vi "Shooter logic.vi"(0 "Low Pressure?":bool, 1 "Fire Main":bool, 2 "Fire 3":bool, 3 "Fire 2":bool, 5 "Grabber Button":bool, 6 "Time Between Open and Shoot":u32=250, 7 "Arms Up button":bool, 8 "Release to Retract":u32=750, 9 "Arms Down Button":bool, 10 "Arms up and down":dbl) -> ()   [LabVIEW 2013]
uses:
  <vilib>/Rock Robotics/WPI/Solenoid/WPI_SolenoidValue.ctl
  <vilib>/Rock Robotics/WPI/Solenoid/WPI_SolenoidSetEnum.vi
  Robot Global Data.vi
panel:
  in  "Bottom Limit":dbl
  in  "Top Limit":dbl
  in  "Potientiometer?":bool
  out "Voltage":dbl
  in  "Arm State":enum16{"Close Arms", "Open Arms"}(ring)
  in  "Launcher State":T1(ring)=enum."Retract"
  out "Tick":u32
  out "Retract Position":T2
  out "Shooter Position":T2
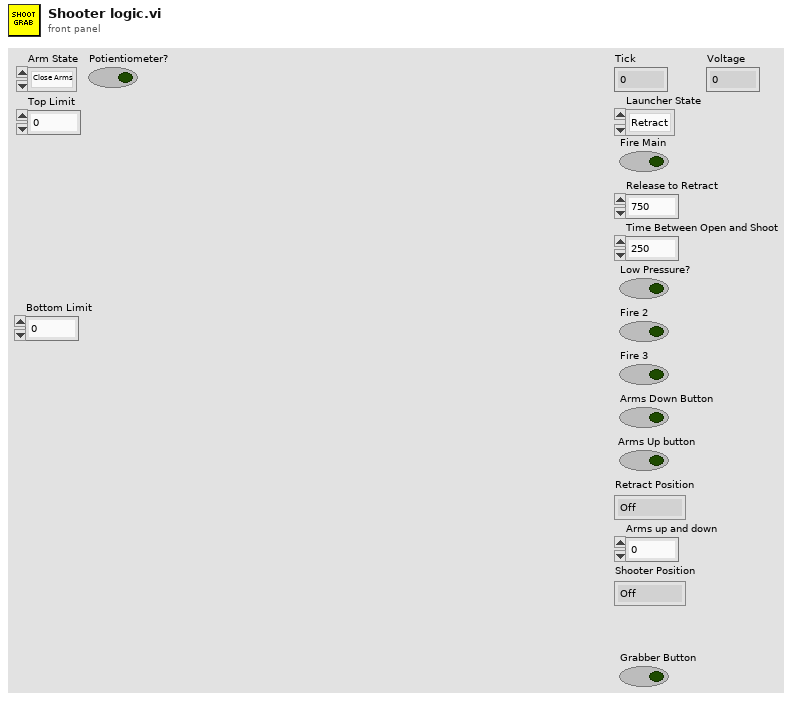
[diagram p1: front panel]
types:
  T1 = enum16{"Open Arms", "Arms Open", "Shoot", "Out", "Retract"}
  T2 = typedef "WPI_SolenoidValue.ctl" = enum16{"Off", "On", "Forward", "Reverse"}
  T3 = typedef "WPI_DigitalInputDevRef.ctl" = cluster{"DevStatus":errorcluster, "DIO Channel":T4, "Digital Module":T5}
  T4 = typedef "FPGA_DIOChannel.ctl" = enum8{"DIO 1", "DIO 2", "DIO 3", "DIO 4", "DIO 5", "DIO 6", "DIO 7", "DIO 8", "DIO 9", "DIO 10", "DIO 11", "DIO 12", "DIO 13", "DIO 14", "Invalid"}
  T5 = typedef "FPGA_TypedefDigitalModule.ctl" = enum16{"Digital Module 1", "Digital Module 2"}
  T6 = typedef "WPI_SolenoidDevRef.ctl" = cluster{"DevStatus":errorcluster, "Solenoid Module":T7, "Forward Solenoid Channel":T8, "Reverse Solenoid Channel":T8}
  T7 = typedef "FPGA_TypedefSolenoidModule.ctl" = enum16{"Solenoid Module 1", "Solenoid Module 2"}
  T8 = typedef "WPI_SolenoidChannel.ctl" = enum8{"Solenoid 1", "Solenoid 2", "Solenoid 3", "Solenoid 4", "Solenoid 5", "Solenoid 6", "Solenoid 7", "Solenoid 8", "Invalid"}
  T9 = typedef "WPI_AnalogChannelDevRef.ctl" = cluster{"DevStatus":errorcluster, "Analog Module":T10, "Analog Channel":T11}
  T10 = typedef "FPGA_TypedefAnalogModule.ctl" = enum16{"Analog Module 1", "Analog Module 2"}
  T11 = typedef "FPGA_AIChannel.ctl" = enum8{"AI 1", "AI 2", "AI 3", "AI 4", "AI 5", "AI 6", "AI 7", "AI 8", "Invalid"}
  T12 = typedef "WPI_MotorControlDeviceRef.ctl" = cluster{"DeviceStatus":errorcluster, "Type":enum16{"PWM", "CAN"}, "PWM":cluster{"Digital Module":T5, "PWM Channel":T13, "DeadBand":T14}, "CAN":cluster{"Device Number":u8, "Control Mode":T15, "Semaphore":T16, "Max Vout":dbl}, "Invert":bool, "TransformRef":T17, "InvTransformRef":T17}
  T13 = typedef "FPGA_DIOPWMChannel.ctl" = enum8{"PWM 1", "PWM 2", "PWM 3", "PWM 4", "PWM 5", "PWM 6", "PWM 7", "PWM 8", "PWM 9", "PWM 10", "Invalid"}
  T14 = typedef "WPI_PWMDeadband.ctl" = cluster{"Name":string, "maxPositivePwm":i32, "minPositivePwm":i32, "centerPwm":i32, "maxNegativePwm":i32, "minNegativePwm":i32, "angularRange":u16}
  T15 = typedef "WPI_CANJaguar_ControlMode.ctl" = enum8{"Percent VBus", "Current", "Speed", "Position", "Voltage"}
  T16 = typedef "Semaphore RefNum" = refnum<k1>
  T17 = typedef "WPI_PWMTransform_ConPane.ctl" = refnum<vi>
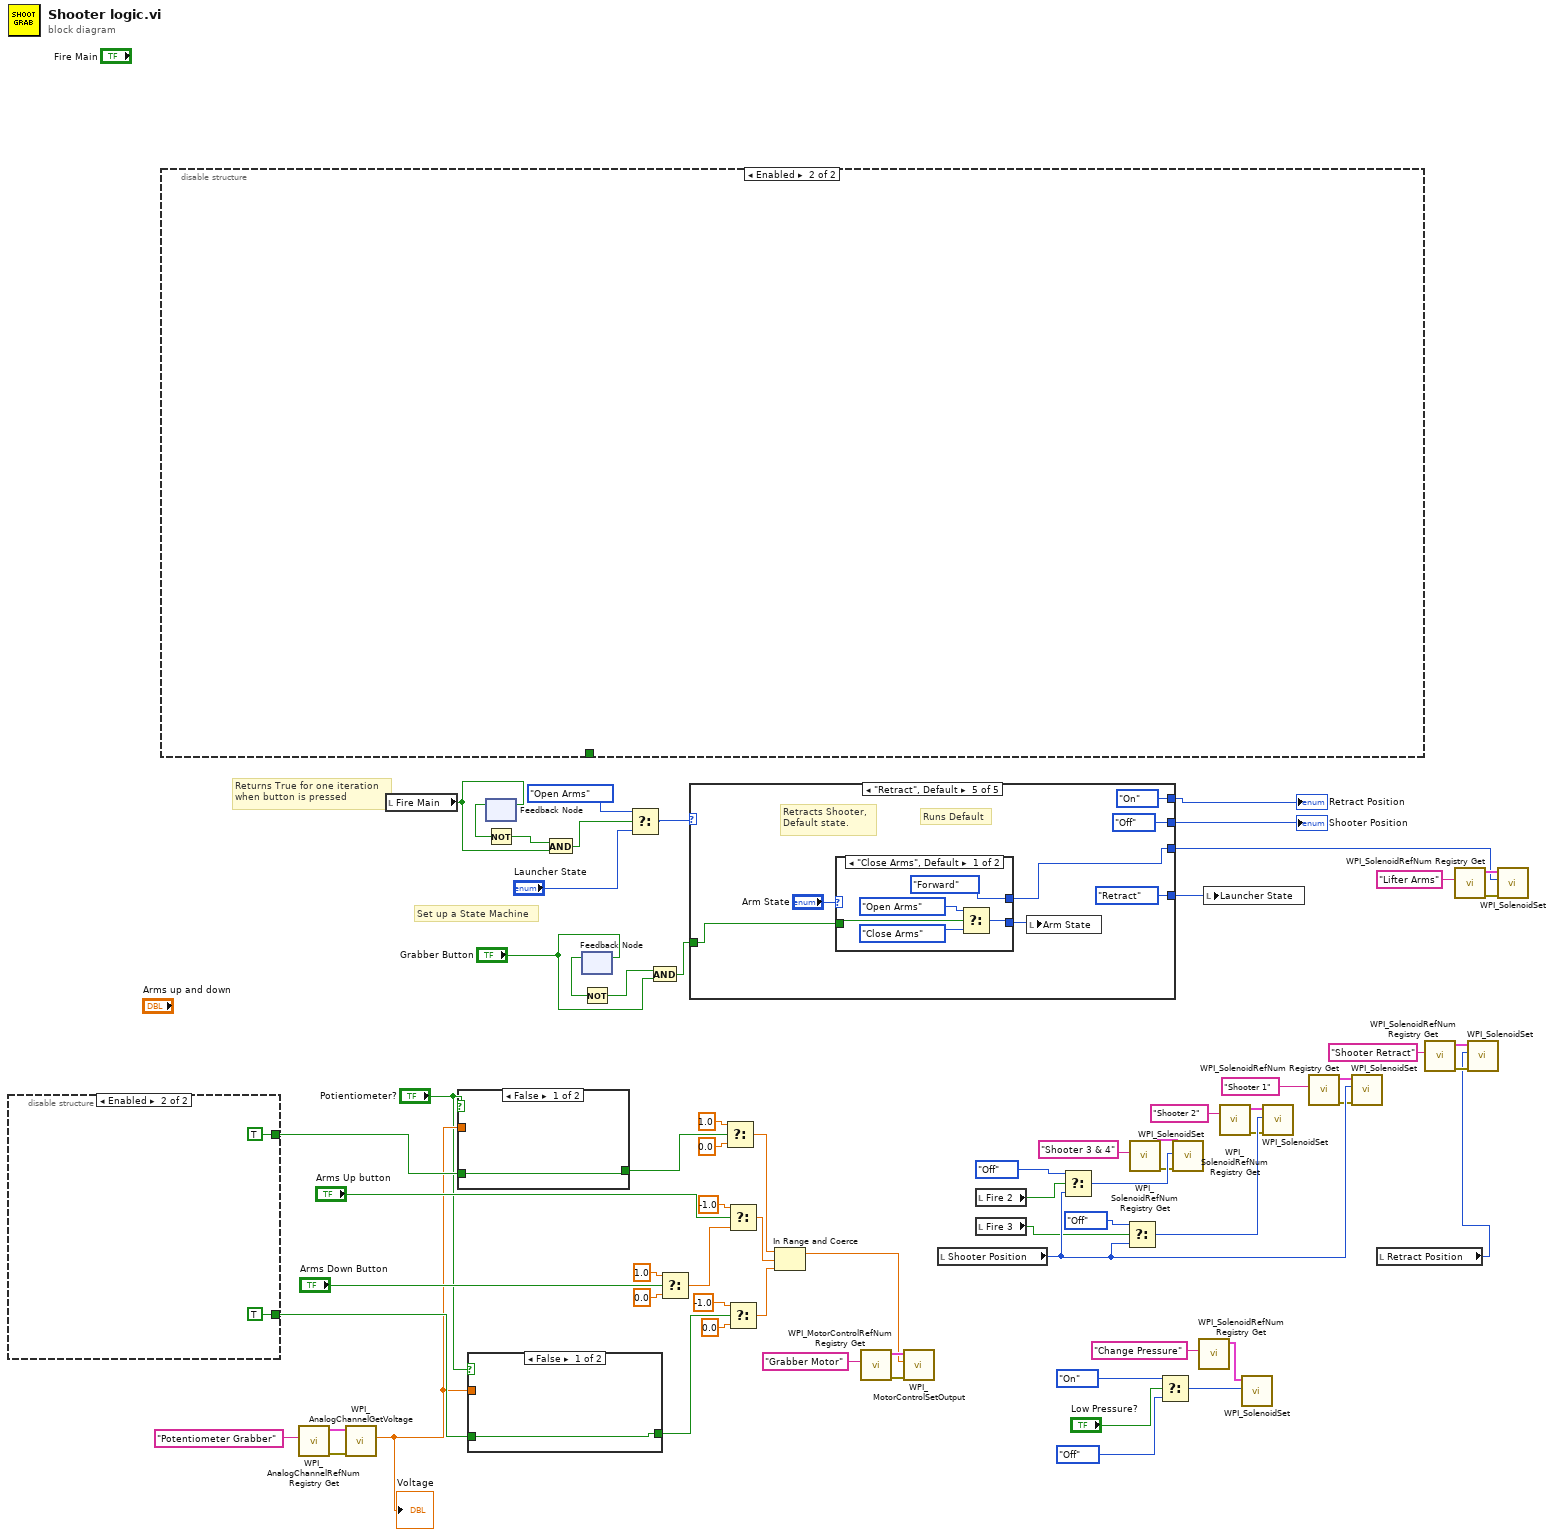
[diagram p0: block diagram]
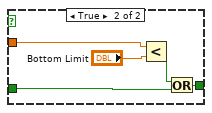
[diagram p2: hidden frame]
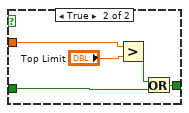
[diagram p3: hidden frame]
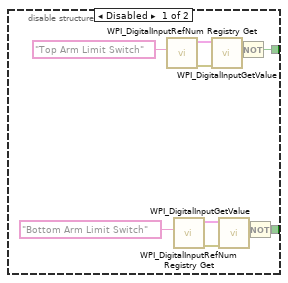
[diagram p4: hidden frame]
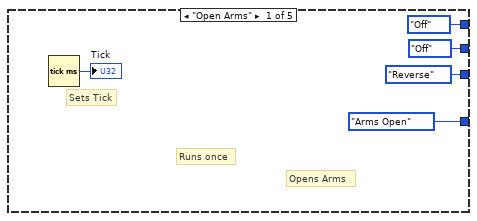
[diagram p5: hidden frame]
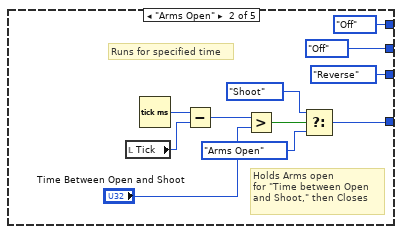
[diagram p6: hidden frame]
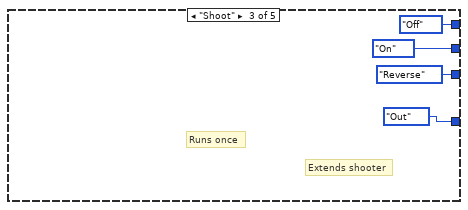
[diagram p7: hidden frame]
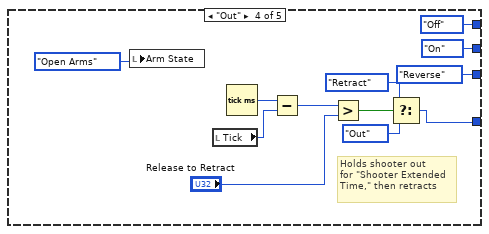
[diagram p8: hidden frame]
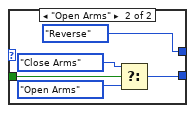
[diagram p9: hidden frame]
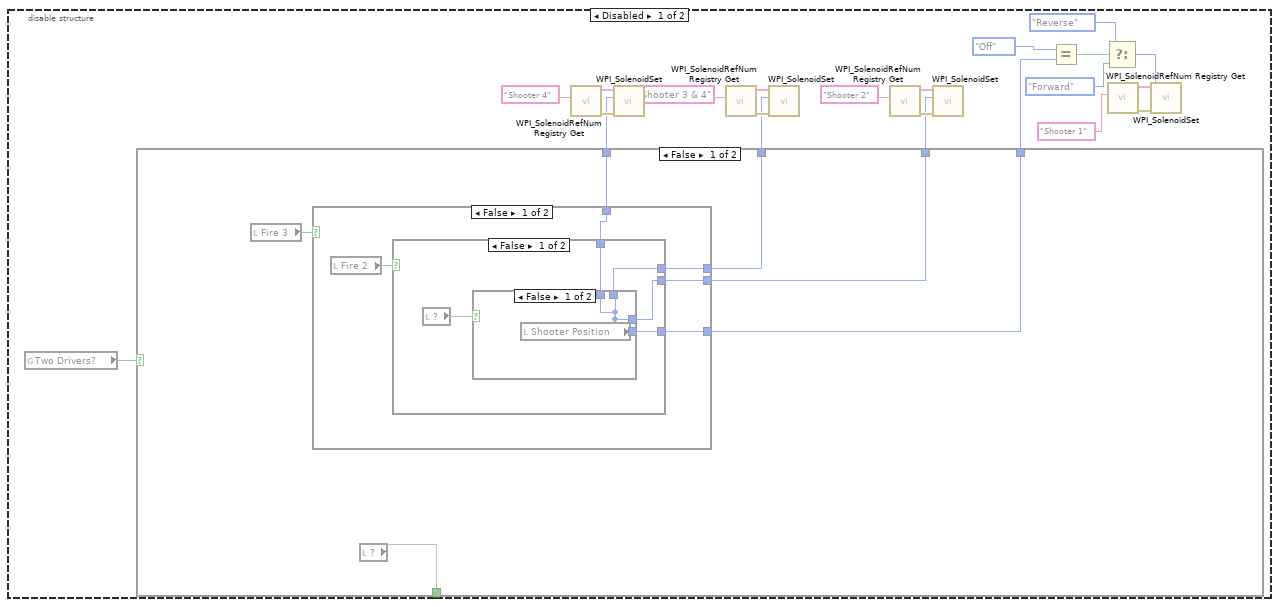
[diagram p10: hidden frame]
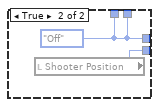
[diagram p11: hidden frame]
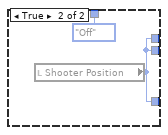
[diagram p12: hidden frame]
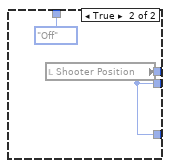
[diagram p13: hidden frame]
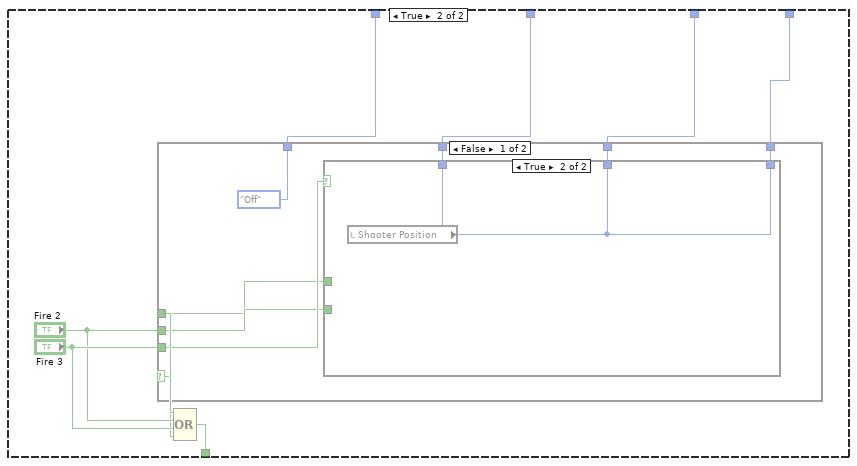
[diagram p14: hidden frame]
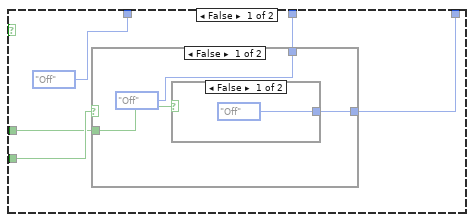
[diagram p15: hidden frame]
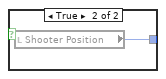
[diagram p16: hidden frame]
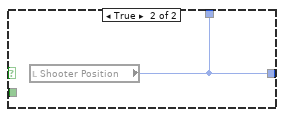
[diagram p17: hidden frame]
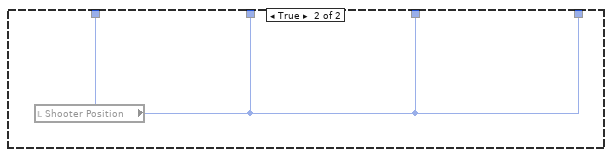
[diagram p18: hidden frame]
diagram:
  # "Set up a State Machine"
  # "Returns True for one iteration\nwhen button is pressed"
  n1 = disable-structure shown="Enabled" {
    disable-tunnel: [w72 TRUE ("Value")] -> w5
    disable-tunnel: [w71 TRUE ("Value")] -> w4
    frame Disabled {
      n2 = call <vilib>:"WPI_DigitalInputRefNum Registry Get.vi"("refnum name"="Top Arm Limit Switch") -> ("error out"=w78:errorcluster, "DigitalInputDevRef"=w79:T3)  [unwired: 9 in]
      n3 = call <vilib>:"WPI_DigitalInputRefNum Registry Get.vi"("refnum name"="Bottom Arm Limit Switch") -> ("error out"=w75:errorcluster, "DigitalInputDevRef"=w76:T3)  [unwired: 9 in]
      n4 = call <vilib>:"WPI_DigitalInputGetValue.vi"("error in (no error)"=w78, "DigitalInputDevRef"=w79) -> ("Value"=w74:bool)  [unwired: 7 in, 2 out]
      n5 = call <vilib>:"WPI_DigitalInputGetValue.vi"("error in (no error)"=w75, "DigitalInputDevRef"=w76) -> ("Value"=w73:bool)  [unwired: 7 in, 2 out]
      n6 = Not(x=w74) -> (.not. x?=w72:bool)
      n7 = Not(x=w73) -> (.not. x?=w71:bool)
    }
    frame Enabled {
    }
  }
  n8 = disable-structure shown="Enabled" {
    disable-tunnel: [w105 _] -> _
    frame Disabled {
      n9 = global read "Robot Global Data.vi" "Two Drivers?"() -> (w104:bool)
      n10 = case shown="False" w104 {
        tunnel: [w111 w137] -> w105
        tunnel: [w106 w132] -> w86
        tunnel: [w109 w131] -> w85
        tunnel: [w108 w130] -> w84
        tunnel: [w107 w129] -> w83
        frame False {
          n11 = local read "Fire 3"() -> (w110:bool)
          n12 = case shown="False" w110 {
            tunnel: [w115 w128] -> w109
            tunnel: [w114 w128] -> w108
            tunnel: [w113 w128] -> w107
            tunnel: [w112 WPI_SolenoidValue."Off" ("Position")] -> w106
            frame False {
              n13 = local read "Fire 2"() -> (w116:bool)
              n14 = case shown="False" w116 {
                tunnel: [w118 w126] -> w115
                tunnel: [w119 w126] -> w114
                tunnel: [w120 w126] -> w113
                tunnel: [w117 WPI_SolenoidValue."Off" ("Position")] -> w112
                frame False {
                  n15 = local read item#-1() -> (w121)
                  n16 = case shown="False" w121 {
                    tunnel: [w122 w124] -> w120
                    tunnel: [w122 w123] -> w119
                    tunnel: [w122 w123] -> w118
                    tunnel: [w122 w123] -> w117
                    frame False {
                      n17 = local read "Shooter Position"() -> (w122:T2)
                    }
                    frame True {
                      w123 = WPI_SolenoidValue."Off" ("Position")
                      n18 = local read "Shooter Position"() -> (w124:T2)
                    }
                  }
                }
                frame True {
                  n19 = local read "Shooter Position"() -> (w126:T2)
                }
              }
            }
            frame True {
              n20 = local read "Shooter Position"() -> (w128:T2)
            }
          }
          n21 = local read item#-1() -> (w111)
        }
        frame True {
          n22 = Compound Arithmetic op=OR("Fire 2", "Fire 3") -> (w137:bool, w134:bool, w133:bool)
          n23 = case shown="False" w133 {
            tunnel: [w140 w157] -> w129
            tunnel: [w141 w157] -> w130
            tunnel: [w142 w157] -> w131
            tunnel: [WPI_SolenoidValue."Off" ("Value") w157] -> w132
            tunnel: "Fire 3" -> [w143 _]
            tunnel: "Fire 2" -> [w139 _]
            tunnel: w134 -> [w138 _]
            frame False {
              n24 = case shown="True" w143 {
                tunnel: [WPI_SolenoidValue."Off" ("Value") w156] -> w142
                tunnel: [w149 w156] -> w141
                tunnel: [w148 w156] -> w140
                tunnel: w139 -> [w147 _]
                tunnel: w138 -> [w146 _]
                frame False {
                  n25 = case shown="False" w147 {
                    tunnel: [WPI_SolenoidValue."Off" ("Value") w155] -> w149
                    tunnel: [w150 w155] -> w148
                    tunnel: w146 -> [w151 _]
                    frame False {
                      n26 = case shown="False" w151 {
                        tunnel: [WPI_SolenoidValue."Off" ("Value") w154] -> w150
                        frame False {
                        }
                        frame True {
                          n27 = local read "Shooter Position"() -> (w154:T2)
                        }
                      }
                    }
                    frame True {
                      n28 = local read "Shooter Position"() -> (w155:T2)
                    }
                  }
                }
                frame True {
                  n29 = local read "Shooter Position"() -> (w156:T2)
                }
              }
            }
            frame True {
              n30 = local read "Shooter Position"() -> (w157:T2)
            }
          }
        }
      }
      n31 = call <vilib>:"WPI_SolenoidRefNum Registry Get.vi"("refnum name"="Shooter 4") -> ("error out"=w96:errorcluster, "SolenoidDevRef"=w97:T6)  [unwired: 9 in]
      n32 = call-poly <vilib>:"WPI_SolenoidSet.vi"("error in (no error)"=w96, "Value"=w86, "SolenoidDevRef"=w97) -> ()  [unwired: 7 in, 2 out]
      n33 = call <vilib>:"WPI_SolenoidRefNum Registry Get.vi"("refnum name"="Shooter 3 & 4") -> ("error out"=w99:errorcluster, "SolenoidDevRef"=w98:T6)  [unwired: 9 in]
      n34 = call-poly <vilib>:"WPI_SolenoidSet.vi"("error in (no error)"=w99, "Value"=w85, "SolenoidDevRef"=w98) -> ()  [unwired: 7 in, 2 out]
      n35 = call <vilib>:"WPI_SolenoidRefNum Registry Get.vi"("refnum name"="Shooter 2") -> ("error out"=w102:errorcluster, "SolenoidDevRef"=w103:T6)  [unwired: 9 in]
      n36 = call-poly <vilib>:"WPI_SolenoidSet.vi"("error in (no error)"=w102, "Value"=w84, "SolenoidDevRef"=w103) -> ()  [unwired: 7 in, 2 out]
      n37 = Equal?(x=WPI_SolenoidValue."Off" ("y"), y=w83) -> (x = y?=w89:bool)
      n38 = Select(t=WPI_SolenoidValue."Reverse" ("y"), s=w89, f=WPI_SolenoidValue."Forward" ("y")) -> (s? t:f=w92:T2)
      n39 = call <vilib>:"WPI_SolenoidRefNum Registry Get.vi"("refnum name"="Shooter 1") -> ("error out"=w88:errorcluster, "SolenoidDevRef"=w87:T6)  [unwired: 9 in]
      n40 = call-poly <vilib>:"WPI_SolenoidSet.vi"("error in (no error)"=w88, "Value"=w92, "SolenoidDevRef"=w87) -> ()  [unwired: 7 in, 2 out]
    }
    frame Enabled {
    }
  }
  n41 = call <vilib>:"WPI_AnalogChannelRefNum Registry Get.vi"("refnum name"="Potentiometer Grabber") -> ("error out"=w21:errorcluster, "AIDeviceRef"=w20:T9)  [unwired: 9 in]
  n42 = call <vilib>:"WPI_AnalogChannelGetVoltage.vi"("error in (no error)"=w21, "AIDeviceRef"=w20) -> ("Voltage"=w2:dbl)  [unwired: 7 in, 2 out]
  "Voltage" <- w2
  n43 = local read "Fire Main"() -> (w36:bool)
  n44 = case shown="False" "Potientiometer?" {
    tunnel: [w158 w161] -> w6
    tunnel: w5 -> [w158 w162]
    tunnel: w2 -> [_ w160]
    frame False {
    }
    frame True {
      n45 = Greater?(x=w160, y="Top Limit") -> (0:w163:bool)
      n46 = Or(x=w163, y=w162) -> (x .or. y?=w161:bool)
    }
  }
  n47 = case shown="False" "Potientiometer?" {
    tunnel: [w164 w167] -> w3
    tunnel: w4 -> [w164 w168]
    tunnel: w2 -> [_ w166]
    frame False {
    }
    frame True {
      n48 = Less?(x=w166, y="Bottom Limit") -> (x < y?=w169:bool)
      n49 = Or(x=w169, y=w168) -> (x .or. y?=w167:bool)
    }
  }
  n50 = feedback #1() -> (w37:bool)  [unwired: 1 in]
  n51 = feedback-in #1(w36) -> ()
  n52 = Not(x=w37) -> (.not. x?=w38:bool)
  n53 = And(x=w38, y=w36) -> (x .and. y?=w33:bool)
  n54 = feedback #2() -> (w25:bool)  [unwired: 1 in]
  n55 = feedback-in #2("Grabber Button") -> ()
  n56 = Not(x=w25) -> (.not. x?=w24:bool)
  n57 = Select(t=T1."Open Arms", s=w33, f="Launcher State") -> (s? t:f=w35:T1)
  n58 = And(x=w24, y="Grabber Button") -> (x .and. y?=w23:bool)
  n59 = Select(t=1.0, s="Arms Down Button", f=0.0) -> (s? t:f=w15:dbl)
  n60 = case shown="\"Retract\", Default" w35 {
    tunnel: [T1."Arms Open" ("Launcher State") w177 T1."Out" ("Launcher State") w195 T1."Retract" ("Launcher State")] -> w27
    tunnel: [WPI_SolenoidValue."Reverse" ("Arm Position") WPI_SolenoidValue."Reverse" ("Arm Position") WPI_SolenoidValue."Reverse" ("Arm Position") WPI_SolenoidValue."Reverse" ("Arm Position") w205] -> w26
    tunnel: [WPI_SolenoidValue."Off" ("Value") WPI_SolenoidValue."Off" ("Value") WPI_SolenoidValue."Off" ("Value") WPI_SolenoidValue."Off" ("Value") WPI_SolenoidValue."On" ("Value")] -> w28
    tunnel: w23 -> [_ _ _ _ w206]
    tunnel: [WPI_SolenoidValue."Off" ("Value") WPI_SolenoidValue."Off" ("Value") WPI_SolenoidValue."On" ("Value") WPI_SolenoidValue."On" ("Value") WPI_SolenoidValue."Off" ("Value")] -> w18
    frame "Open Arms" {
      # "Opens Arms"
      # "Runs once"
      # "Sets Tick"
      n61 = Tick Count (ms)() -> (millisecond timer value=→"Tick":u32)
    }
    frame "Arms Open" {
      # "Runs for specified time"
      # "Holds Arms open\nfor \"Time between Open\nand Shoot,\" then Closes"
      n62 = local read "Tick"() -> (w184:u32)
      n63 = Tick Count (ms)() -> (millisecond timer value=w185:u32)
      n64 = Subtract(x=w185, y=w184) -> (x-y=w183:u32)
      n65 = Greater?(x=w183, y="Time Between Open and Shoot") -> (0:w182:bool)
      n66 = Select(t=T1."Shoot" ("Launcher State"), s=w182, f=T1."Arms Open" ("Launcher State")) -> (s? t:f=w177:T1)
    }
    frame "Shoot" {
      # "Runs once"
      # "Extends shooter"
    }
    frame "Out" {
      # "Holds shooter out\nfor \"Shooter Extended\nTime,\" then retracts"
      n67 = local write "Arm State"(enum16{"Close Arms", "Open Arms"}."Open Arms" ("Arm State")) -> ()
      n68 = local read "Tick"() -> (w200:u32)
      n69 = Tick Count (ms)() -> (millisecond timer value=w201:u32)
      n70 = Subtract(x=w201, y=w200) -> (x-y=w199:u32)
      n71 = Greater?(x=w199, y="Release to Retract") -> (0:w198:bool)
      n72 = Select(t=T1."Retract" ("Launcher State"), s=w198, f=T1."Out" ("Launcher State")) -> (s? t:f=w195:T1)
    }
    frame "Retract", Default {
      # "Runs Default"
      # "Retracts Shooter, \nDefault state."
      n73 = case shown="\"Close Arms\", Default" "Arm State" {
        tunnel: w206 -> [w209 w214]
        tunnel: [WPI_SolenoidValue."Forward" ("Value") WPI_SolenoidValue."Reverse" ("Value")] -> w205
        tunnel: [w210 w215] -> w203
        frame "Close Arms", Default {
          n74 = Select(t=enum16{"Close Arms", "Open Arms"}."Open Arms", s=w209, f=enum16{"Close Arms", "Open Arms"}."Close Arms") -> (s? t:f=w210:enum16{"Close Arms", "Open Arms"})
        }
        frame "Open Arms" {
          n75 = Select(t=enum16{"Close Arms", "Open Arms"}."Close Arms", s=w214, f=enum16{"Close Arms", "Open Arms"}."Open Arms") -> (s? t:f=w215:enum16{"Close Arms", "Open Arms"})
        }
      }
      n76 = local write "Arm State"(w203) -> ()
    }
  }
  "Shooter Position" <- w18
  "Retract Position" <- w28
  n77 = Select(t=1.0, s=w6, f=0.0) -> (s? t:f=w10:dbl)
  n78 = Select(t=-1.0, s="Arms Up button", f=w15) -> (s? t:f=w13:dbl)
  n79 = Select(t=-1.0, s=w3, f=0.0) -> (s? t:f=w7:dbl)
  n80 = In Range and Coerce(upper limit=w10, x=w13, lower limit=w7) -> (coerced(x)=w29:dbl)  [unwired: 1 out]
  n81 = call <vilib>:"WPI_MotorControlRefNum Registry Get.vi"("refnum name"="Grabber Motor") -> ("error out"=w41:errorcluster, "MotorControlDevRef"=w40:T12)  [unwired: 9 in]
  n82 = call <vilib>:"WPI_MotorControlSetOutput.vi"("error in (no error)"=w41, "Output"=w29, "MotorControlDevRef"=w40) -> ()  [unwired: 6 in, 3 out]
  n83 = local read "Shooter Position"() -> (w67:T2)
  n84 = local read "Fire 2"() -> (w62:bool)
  n85 = local read "Fire 3"() -> (w58:bool)
  n86 = Select(t=WPI_SolenoidValue."Off", s=w62, f=w67) -> (s? t:f=w63:T2)
  n87 = Select(t=WPI_SolenoidValue."Off", s=w58, f=w67) -> (s? t:f=w59:T2)
  n88 = call <vilib>:"WPI_SolenoidRefNum Registry Get.vi"("refnum name"="Shooter 3 & 4") -> ("error out"=w53:errorcluster, "SolenoidDevRef"=w54:T6)  [unwired: 9 in]
  n89 = Select(t=WPI_SolenoidValue."On", s="Low Pressure?", f=WPI_SolenoidValue."Off" ("t")) -> (s? t:f=w44:T2)
  n90 = call-poly <vilib>:"WPI_SolenoidSet.vi"("error in (no error)"=w53, "Value"=w63, "SolenoidDevRef"=w54) -> ()  [unwired: 7 in, 2 out]
  n91 = call <vilib>:"WPI_SolenoidRefNum Registry Get.vi"("refnum name"="Change Pressure") -> ("SolenoidDevRef"=w48:T6)  [unwired: 9 in, 1 out]
  n92 = local write "Launcher State"(w27) -> ()
  n93 = call <vilib>:"WPI_SolenoidRefNum Registry Get.vi"("refnum name"="Shooter 2") -> ("error out"=w50:errorcluster, "SolenoidDevRef"=w49:T6)  [unwired: 9 in]
  n94 = call-poly <vilib>:"WPI_SolenoidSet.vi"("Value"=w44, "SolenoidDevRef"=w48) -> ()  [unwired: 8 in, 2 out]
  n95 = call-poly <vilib>:"WPI_SolenoidSet.vi"("error in (no error)"=w50, "Value"=w59, "SolenoidDevRef"=w49) -> ()  [unwired: 7 in, 2 out]
  n96 = call <vilib>:"WPI_SolenoidRefNum Registry Get.vi"("refnum name"="Shooter 1") -> ("error out"=w56:errorcluster, "SolenoidDevRef"=w57:T6)  [unwired: 9 in]
  n97 = call-poly <vilib>:"WPI_SolenoidSet.vi"("error in (no error)"=w56, "Value"=w67, "SolenoidDevRef"=w57) -> ()  [unwired: 7 in, 2 out]
  n98 = local read "Retract Position"() -> (w42:T2)
  n99 = call <vilib>:"WPI_SolenoidRefNum Registry Get.vi"("refnum name"="Shooter Retract") -> ("error out"=w65:errorcluster, "SolenoidDevRef"=w64:T6)  [unwired: 9 in]
  n100 = call <vilib>:"WPI_SolenoidRefNum Registry Get.vi"("refnum name"="Lifter Arms") -> ("error out"=w69:errorcluster, "SolenoidDevRef"=w68:T6)  [unwired: 9 in]
  n101 = call-poly <vilib>:"WPI_SolenoidSet.vi"("error in (no error)"=w65, "Value"=w42, "SolenoidDevRef"=w64) -> ()  [unwired: 7 in, 2 out]
  n102 = call-poly <vilib>:"WPI_SolenoidSet.vi"("error in (no error)"=w69, "Value"=w26, "SolenoidDevRef"=w68) -> ()  [unwired: 7 in, 2 out]
